vi "Main.vi"() -> ()   [LabVIEW 2019]
doc: "This template is for the Queued Message Handler design pattern.\n\nThe Event Handling Loop generates messages based on user interface actions.\n\nThe Message Handling Loop processes messages generated by the Event Handling Loop, or by other messages. The messages are string values, so new messages can be added easily to the Message Cases case structure in the Message Handling Loop. Each message cluster can also provide an optional value for Message Data, which is a variant that can be converted to whatever message-specific data is required."
uses:
  controls/Main UI Data.ctl
  support/Message Queue/Enqueue Message (Single).vi
  <vilib>/Utility/error.llb/Error Cluster From Error Code.vi
  <vilib>/ErrorRing/Error Ring.xnode
  support/Message Queue/Message Named Queue.lvlib
  support/User Event - Stop/User Event - Stop.lvlib
panel:
  out "Display <Replace Me> 2":string
  in  "Hamburger Menu Button":bool
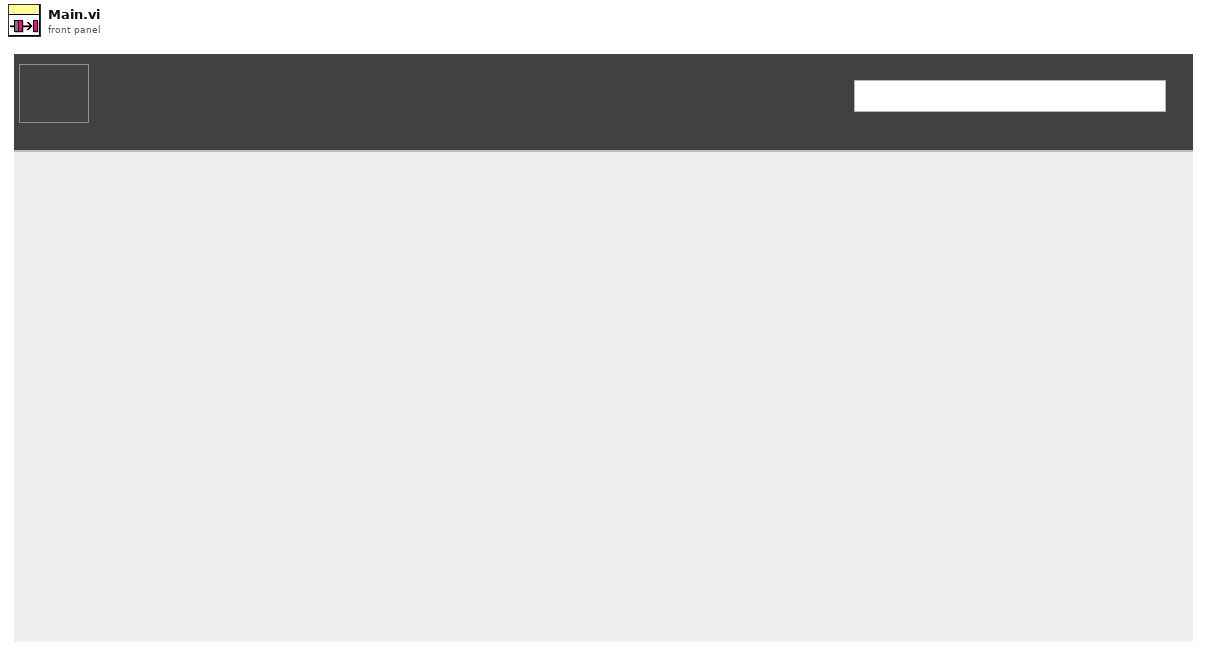
[diagram p1: front panel]
types:
  T1 = typedef "Main UI Data.ctl" = cluster{"Replace me":string}
  T2 = typedef "Message Named Queue.lvlib/All Message Queues.ctl" = cluster{"Main UI":refnum<queue>, "Hamburger UI":refnum<queue>}
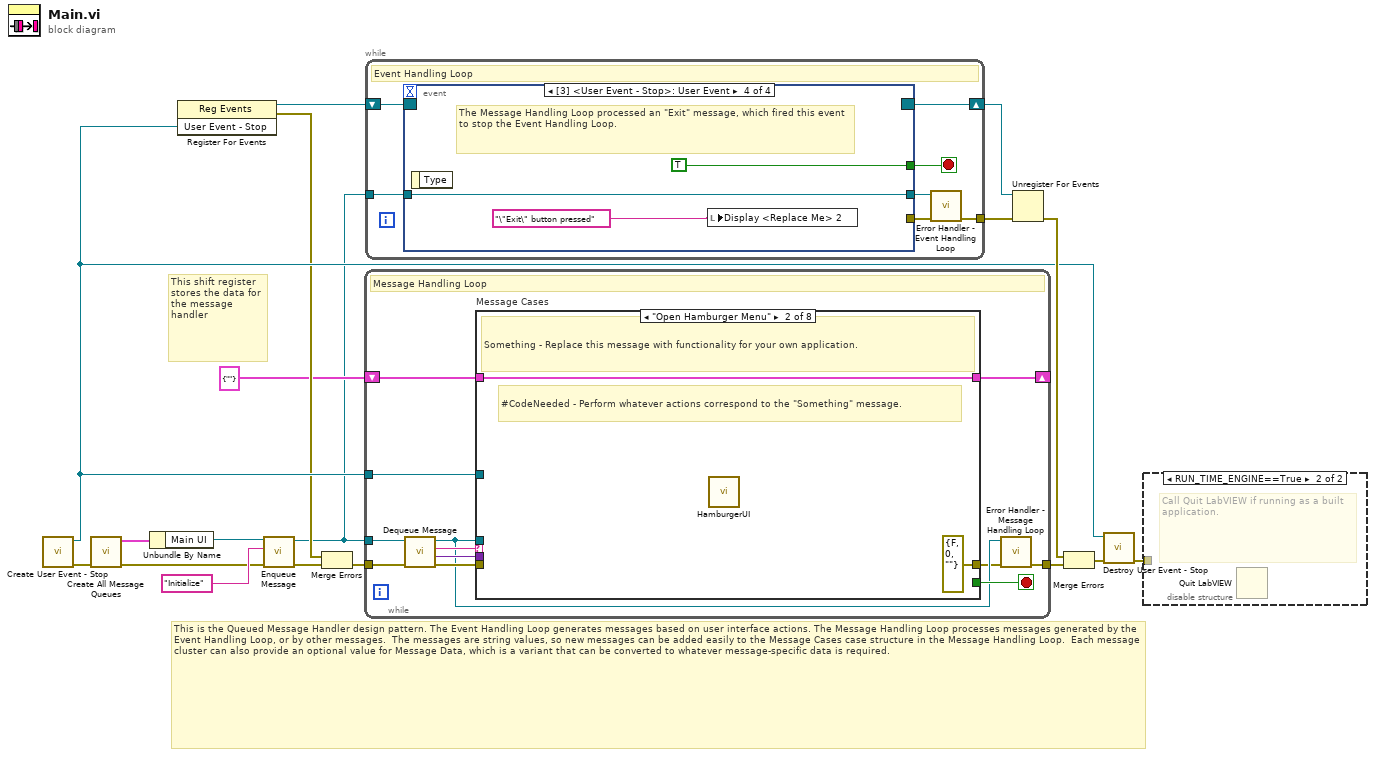
[diagram p0: block diagram]
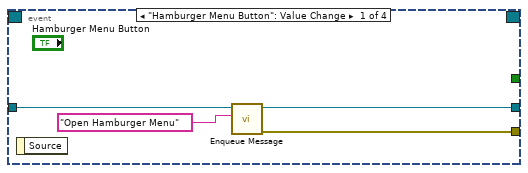
[diagram p3: hidden frame]
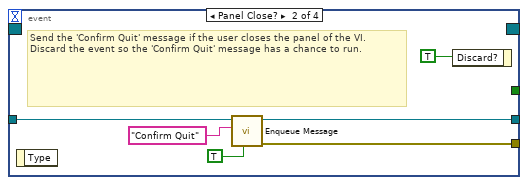
[diagram p4: hidden frame]
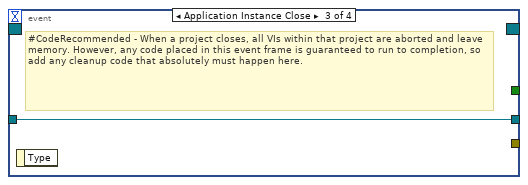
[diagram p5: hidden frame]
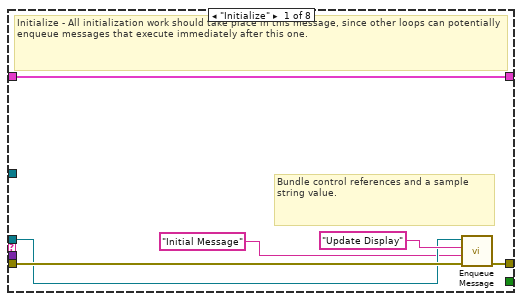
[diagram p6: hidden frame]
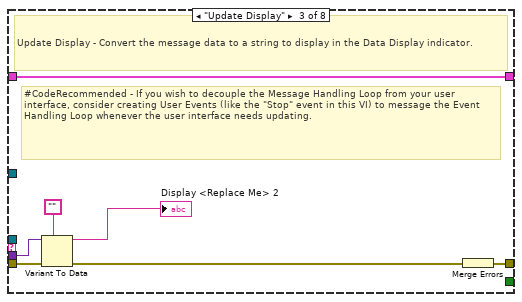
[diagram p7: hidden frame]
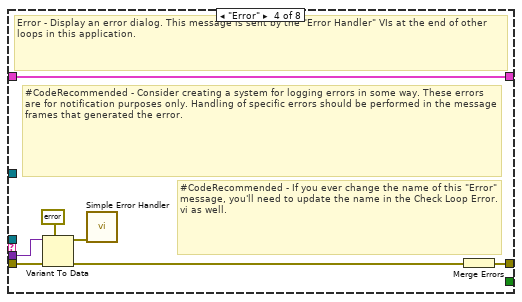
[diagram p8: hidden frame]
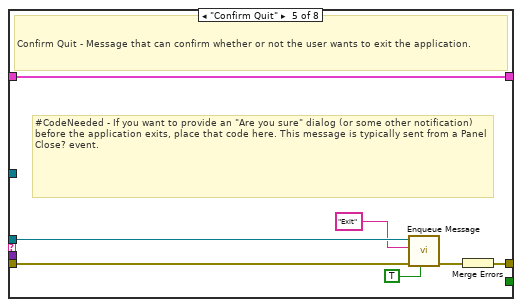
[diagram p9: hidden frame]
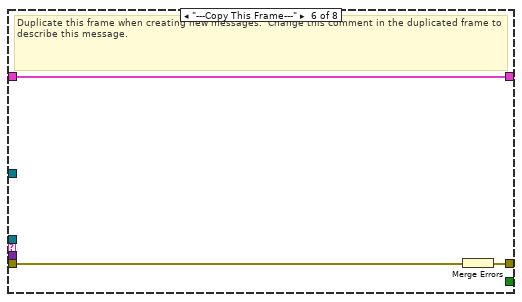
[diagram p10: hidden frame]
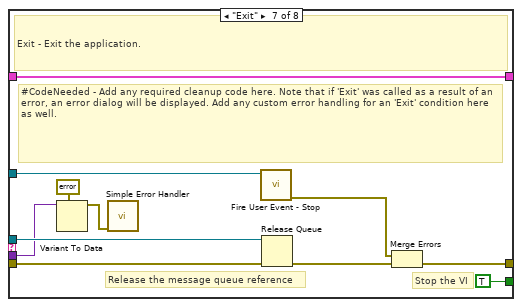
[diagram p11: hidden frame]
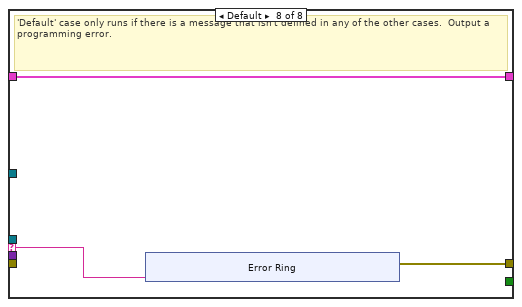
[diagram p12: hidden frame]
diagram:
  # "This is the Queued Message Handler design pattern. The Event Handling Loop generates messages based on user interface actions. The Message Handling Loop processes messages generated by the Event Handling Loop, or by other messages.  The messages are string values, so new messages can be added easily to the Message Cases case structure in the Message Handling Loop.  Each message cluster can also provide an optional value for Message Data, which is a variant that can be converted to whatever message-specific data is required."
  # "This shift register stores the data for the message handler"
  n1 = call "Create User Event - Stop.vi"() -> ("error out"=w16:errorcluster, "User Event - Stop"=w9:refnum<user-event>)  [unwired: 10 in]
  n2 = call "Create All Message Queues.vi"("error in (no error)"=w16) -> ("error out"=w1:errorcluster, "Message Queues out"=w18:T2)  [unwired: 9 in]
  n3 = Unbundle By Name(w18) -> ("Main UI"=w4:refnum<queue>)
  n4 = register-events(w9) -> (reference out=w10:refnum<event-registration>, error out=w7:errorcluster)  [unwired: 2 in]
  n5 = call-poly "Enqueue Message.vi"("error in (no error)"=w1, "Message"="Initialize", "Message Queue"=w4) -> ("error out"=w2:errorcluster, "dup Message Queue"=w3:refnum<queue>)  [unwired: 7 in]
  n6 = Merge Errors(w7, w2) -> (w8:errorcluster)
  n7 = while {
    tunnel: w3 -> [w22]
    shift-right: [w29] -> _
    shift-left: T1 {"Replace me"=""} ("Cluster") -> [w30]
    tunnel: w9 -> [w27]
    tunnel: w8 -> [w26]
    tunnel: [w20] -> w17
    stop <- w28 stop-if-true
    # "Message Handling Loop"
    n8 = call "Dequeue Message.vi"("error in (no error)"=w26, "Message Queue"=w22) -> ("error out"=w25:errorcluster, "Message Data"=w23:variant, "Message"=w24:string, "dup Message Queue"=w21:refnum<queue>)  [unwired: 6 in]
    n9 = case "Message Cases" shown="\"Open Hamburger Menu\"" w24 {
      selector: w24 -> [_ _ _ _ _ _ _ w74]
      tunnel: w21 -> [w33 _ _ _ w55 _ w73 _]
      tunnel: w25 -> [w35 _ w43 w52 w59 w62 w66 _]
      tunnel: [w36 errorcluster {"status"=FALSE, "code"=0, "source"=""} ("error out") w44 w46 w57 w60 w69 w75] -> w19
      tunnel: w30 -> [w31 w38 w45 w51 w58 w61 w72 w76]
      tunnel: [w31 w38 w45 w51 w58 w61 w72 w76] -> w29
      tunnel: [_ _ _ _ _ _ TRUE _] -> w28
      tunnel: w23 -> [_ _ w42 w50 _ _ w63 _]
      tunnel: w27 -> [_ _ _ _ _ _ w68 _]
      frame "Initialize" {
        # "Bundle control references and a sample string value."
        # "Initialize - All initialization work should take place in this message, since other loops can potentially enqueue messages that execute immediately after this one."
        n10 = call-poly "Enqueue Message.vi"("error in (no error)"=w35, "Message Data"="Initial Message" ("Initial Message"), "Message"="Update Display", "Message Queue"=w33) -> ("error out"=w36:errorcluster)  [unwired: 6 in, 1 out]
      }
      frame "Open Hamburger Menu" {
        # "#CodeNeeded - Perform whatever actions correspond to the \"Something\" message."
        # "Something - Replace this message with functionality for your own application."
        n11 = call "HamburgerUI.vi"() -> ()  [unwired: 12 in]
      }
      frame "Update Display" {
        # "#CodeRecommended - If you wish to decouple the Message Handling Loop from your user interface, consider creating User Events (like the \"Stop\" event in this VI) to message the Event Handling Loop whenever the user interface needs updating."
        # "Update Display - Convert the message data to a string to display in the Data Display indicator."
        n12 = Variant To Data(error in=w43, type="", Variant=w42) -> (data=→"Display <Replace Me> 2":string, error out=w40:errorcluster)
        n13 = Merge Errors(w40) -> (w44:errorcluster)
      }
      frame "Error" {
        # "#CodeRecommended - If you ever change the name of this \"Error\" message, you'll need to update the name in the Check Loop Error.vi as well."
        # "#CodeRecommended - Consider creating a system for logging errors in some way. These errors are for notification purposes only. Handling of specific errors should be performed in the message frames that generated the error."
        # "Error - Display an error dialog. This message is sent by the \"Error Handler\" VIs at the end of other loops in this application."
        n14 = Variant To Data(error in=w52, type=errorcluster {"status"=FALSE, "code"=0, "source"=""} ("error constant"), Variant=w50) -> (data=w48:errorcluster, error out=w47:errorcluster)
        n15 = call <vilib>:"Simple Error Handler.vi"("error in (no error)"=w48) -> ()  [unwired: 4 in, 5 out]
        n16 = Merge Errors(w47) -> (w46:errorcluster)
      }
      frame "Confirm Quit" {
        # "#CodeNeeded - If you want to provide an \"Are you sure\" dialog (or some other notification) before the application exits, place that code here. This message is typically sent from a Panel Close? event."
        # "Confirm Quit - Message that can confirm whether or not the user wants to exit the application."
        n17 = call-poly "Enqueue Message.vi"("Priority Message? (F)"=TRUE, "error in (no error)"=w59, "Message"="Exit", "Message Queue"=w55) -> ("error out"=w56:errorcluster)  [unwired: 6 in, 1 out]
        n18 = Merge Errors(w56) -> (w57:errorcluster)
      }
      frame "---Copy This Frame---" {
        # "Duplicate this frame when creating new messages.  Change this comment in the duplicated frame to describe this message."
        n19 = Merge Errors(w62) -> (w60:errorcluster)
      }
      frame "Exit" {
        # "Stop the VI"
        # "Release the message queue reference"
        # "#CodeNeeded - Add any required cleanup code here. Note that if 'Exit' was called as a result of an error, an error dialog will be displayed. Add any custom error handling for an 'Exit' condition here as well."
        # "Exit - Exit the application."
        n20 = Variant To Data(type=errorcluster {"status"=FALSE, "code"=0, "source"=""} ("error constant"), Variant=w63) -> (data=w64:errorcluster)  [unwired: 1 in, 1 out]
        n21 = call <vilib>:"Simple Error Handler.vi"("error in (no error)"=w64) -> ()  [unwired: 4 in, 5 out]
        n22 = call "Fire User Event - Stop.vi"("User Event - Stop"=w68) -> ("error out"=w67:errorcluster)  [unwired: 10 in]
        n23 = Release Queue(queue=w73, error in (no error)=w66) -> (error out=w70:errorcluster)  [unwired: 1 in, 2 out]
        n24 = Merge Errors(w67, w70) -> (w69:errorcluster)
      }
      frame Default {
        # "'Default' case only runs if there is a message that isn't defined in any of the other cases.  Output a programming error."
        n25 = xnode "Error Ring"("parameter 0"=w74) -> ("error out"=w75:errorcluster)
      }
    }
    n26 = call "Error Handler - Message Handling Loop.vi"("error in (no error)"=w19, "Message Queue"=w21) -> ("dup error in"=w20:errorcluster)  [unwired: 8 in, 1 out]
  }
  n27 = while {
    tunnel: w3 -> [w90]
    shift-right: [w88] -> w13
    shift-left: w10 -> [w89]
    tunnel: [w84] -> w11
    stop <- w86 stop-if-true
    # "Event Handling Loop"
    n28 = event shown="[3] <User Event - Stop>: User Event" {
      selector: w89 -> [_ _ _ _]
      dyn-events: [_ _ _ _] -> w88
      timeout: _ -> [_ _ _ _]
      tunnel: [_ _ _ TRUE ("Discard?")] -> w86
      tunnel: w90 -> [w94 w99 w101 w104]
      tunnel: [w91 w98 _ _] -> w87
      tunnel: [w93 w97 w101 w104] -> w85
      event "Hamburger Menu Button": Value Change {
        n29 = event-data() -> ()  [unwired: 1 in, 1 out]
        n30 = call-poly "Enqueue Message.vi"("Message"="Open Hamburger Menu", "Message Queue"=w94) -> ("error out"=w91:errorcluster, "dup Message Queue"=w93:refnum<queue>)  [unwired: 8 in]
      }
      event Panel Close? {
        # "Send the 'Confirm Quit' message if the user closes the panel of the VI. Discard the event so the 'Confirm Quit' message has a chance to run."
        n31 = event-data() -> ()  [unwired: 1 in, 1 out]
        n32 = call-poly "Enqueue Message.vi"("Priority Message? (F)"=TRUE, "Message"="Confirm Quit", "Message Queue"=w99) -> ("error out"=w98:errorcluster, "dup Message Queue"=w97:refnum<queue>)  [unwired: 7 in]
        n33 = event-data("Discard?"=TRUE) -> ()  [unwired: 1 in, 1 out]
      }
      event Application Instance Close {
        # "#CodeRecommended - When a project closes, all VIs within that project are aborted and leave memory. However, any code placed in this event frame is guaranteed to run to completion, so add any cleanup code that absolutely must happen here."
        n34 = event-data() -> ()  [unwired: 1 in, 1 out]
      }
      event User Event {
        # "The Message Handling Loop processed an \"Exit\" message, which fired this event to stop the Event Handling Loop."
        n35 = event-data() -> ()  [unwired: 1 in, 1 out]
        n36 = local write "Display <Replace Me> 2"("\"Exit\" button pressed" ("VI Stopped")) -> ()
      }
    }
    n37 = call "Error Handler - Event Handling Loop.vi"("error in (no error)"=w87, "Message Queue"=w85) -> ("dup error in"=w84:errorcluster)  [unwired: 8 in, 1 out]
  }
  n38 = Unregister For Events(event registration refnum=w13, error in=w11) -> (error out=w14:errorcluster)
  n39 = Merge Errors(w14, w17) -> (w15:errorcluster)
  n40 = call "Destroy User Event - Stop.vi"("error in (no error)"=w15, "User Event - Stop"=w9) -> ("error out"=w12:errorcluster)  [unwired: 9 in]
  n41 = disable-structure shown="RUN_TIME_ENGINE==True" {
    disable-tunnel: w12 -> [_ _]
    frame condition #0 (active) {
    }
    frame condition #1 {
      # "Call Quit LabVIEW if running as a built application."
      n42 = Quit LabVIEW() -> ()  [unwired: 1 in]
    }
  }
